vi "Handle Notification.vi"(8 "error in (no error)":errorcluster, 9 "Payload":string, 10 "Notification Type":string, 11 "Power Spectrum Density in":refnum<class "Power Spectrum Density.lvclass">) -> (0 "error out":errorcluster, 3 "Power Spectrum Density out":refnum<class "Power Spectrum Density.lvclass">)   [LabVIEW 2023, in "Power Spectrum Density.lvlib" / "Power Spectrum Density.lvclass"]
uses:
  Power Spectrum Density.lvclass
  Power Spectrum Density.lvclass/Power Spectrum Density.ctl
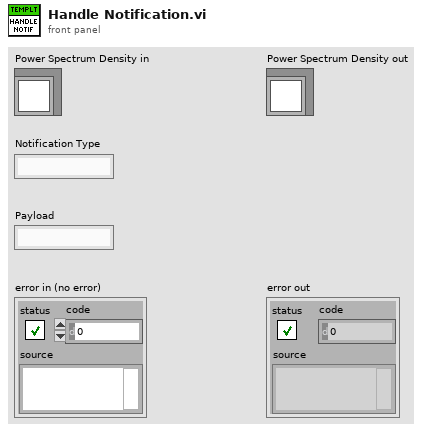
[diagram p1: front panel]
types:
  T1 = typedef "Power Spectrum Density.lvlib/Power Spectrum Density.lvclass/Power Spectrum Density Data.ctl" = cluster{"First Time":bool, "Show PSD Window":bool, "Show PSD Window Clicked":bool, "Export mode":T2, "Window":T3, "dB":bool, "Averaging parameters":cluster{"averaging mode":enum16{"No averaging", "Vector averaging", "RMS averaging", "Peak hold"}, "weighting mode":enum16{"Linear", "Exponential"}, "number of averages":u32}, "Window parameter":dbl, "PSD VI Ref":refnum<vi>}
  T2 = typedef "NI_MAPro.lvlib/Power Spectrum and PSD Export Mode.ctl" = u16
  T3 = typedef "NI_AALPro.lvlib/windowTd.ctl" = u32
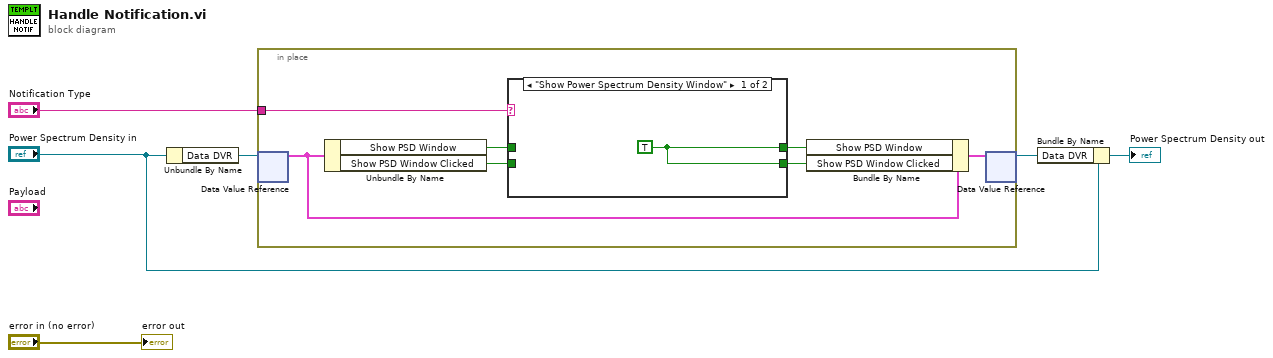
[diagram p0: block diagram]
diagram:
  n1 = Unbundle By Name("Power Spectrum Density in") -> ("Data DVR"=w6:refnum<data-value>)
  n2 = in-place {
    in-place-border: "Notification Type" -> [w13]
    n3 = in-place-dvr #1(w6) -> (w10:T1)  [unwired: 1 out]
    n4 = Unbundle By Name(w10) -> ("Show PSD Window"=w12:bool, "Show PSD Window Clicked"=w11:bool)
    n5 = case shown="\"Show Power Spectrum Density Window\"" w13 {
      tunnel: [w14 w16] -> w9
      tunnel: w12 -> [_ w16]
      tunnel: w11 -> [_ w15]
      tunnel: [w14 w15] -> w8
      frame "Show Power Spectrum Density Window" {
        w14 = TRUE
      }
      frame Default {
      }
    }
    n6 = Bundle By Name(cluster=w10, "Show PSD Window"=w9, "Show PSD Window Clicked"=w8) -> (w7:T1)
    n7 = in-place-dvr #1(w7) -> (w5:refnum<data-value>)  [unwired: 1 out]
  }
  n8 = Bundle By Name(cluster="Power Spectrum Density in", "Data DVR"=w5) -> (→"Power Spectrum Density out":refnum<class "Power Spectrum Density.lvclass">)
  "error out" <- "error in (no error)"
